vi "ReadTimeStamp.vi"(8 "error in":errorcluster, 11 "task/channels in":refnum<k21>) -> (0 "error out":errorcluster, 2 "data":u32, 3 "task out":refnum<k21>)   [LabVIEW 2014]
uses:
  <vilib>/DAQmx/read.llb/DAQmx Read (Counter U32 1Chan 1Samp).vi
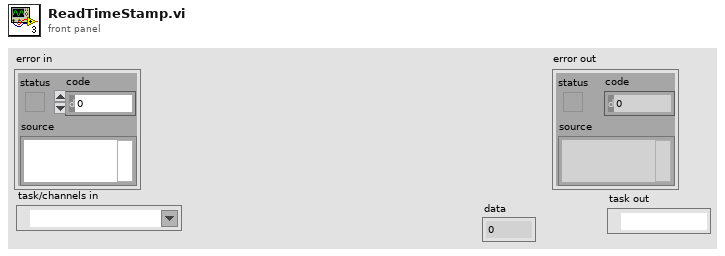
[diagram p1: front panel]
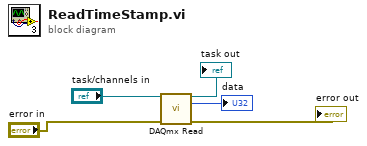
[diagram p0: block diagram]
diagram:
  n1 = call-poly <vilib>:"DAQmx Read.vi"("task/channels in"="task/channels in", "error in"="error in") -> ("task out"=→"task out":refnum<k21>, "data"=→"data":u32, "error out"=→"error out":errorcluster)  [unwired: 11 in]
